vi "Serch.vi"(2 "静态VI":refnum<vi>, 3 "子面板":refnum<vi>) -> ()   [LabVIEW 2015]
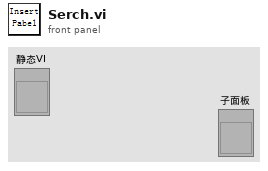
[diagram p1: front panel]
types:
  T1 = enum32{"Bad", "Idle", "Run top level", "Running"}
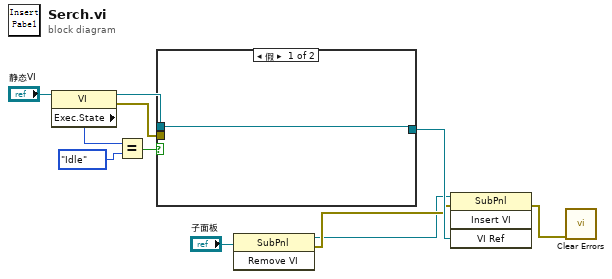
[diagram p0: block diagram]
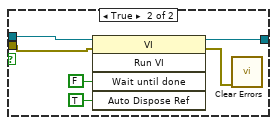
[diagram p2: hidden frame]
diagram:
  n1 = property class="VI"(reference="静态VI") -> (reference out=w1:refnum<vi>, error out=w10:errorcluster, "Exec.State"=w7:T1)  [unwired: 1 in]
  n2 = Equal?(x=w7, y=T1."Idle") -> (x = y?=w9:bool)
  n3 = case shown="假" w9 {
    tunnel: w1 -> [w12 w18]
    tunnel: w10 -> [_ w15]
    tunnel: [w12 w13] -> w11
    frame False {
    }
    frame True {
      n4 = invoke class="VI" method="Run VI"(reference=w18, error in=w15, "Wait until done"=FALSE ("结束前等待"), "Auto Dispose Ref"=TRUE ("自动销毁引用")) -> (reference out=w13:refnum<vi>, error out=w14:errorcluster)  [unwired: 1 in, 3 out]
      n5 = call <vilib>:"Clear Errors.vi"("error in (no error)"=w14) -> ()  [unwired: 5 in, 2 out]
    }
  }
  n6 = invoke class="SubPnl" method="Remove VI"(reference="子面板") -> (reference out=w5:refnum<vi>, error out=w6:errorcluster)  [unwired: 2 in, 1 out]
  n7 = invoke class="SubPnl" method="Insert VI"(reference=w5, error in=w6, "VI Ref"=w11) -> (error out=w2:errorcluster)  [unwired: 1 in, 3 out]
  n8 = call <vilib>:"Clear Errors.vi"("error in (no error)"=w2) -> ()  [unwired: 5 in, 2 out]
